vi "Main Tclk.vi"() -> ()   [LabVIEW 2018] (continued)
                        n3579 = local read "BD1 high limit array"() -> (w9160:sgl[])
                        n3580 = local read "Beam Dump 1 (nA)"() -> (w9152:sgl)
                        n3581 = local read "BD1 low limit array"() -> (w9156:sgl[])
                        n3582 = In Range and Coerce(upper limit=w9153, x=w9152, lower limit=w9154) -> (In Range?=w9163:bool)  [unwired: 1 out]
                        n3583 = Build Array (concatenate)(w9160, w9153) -> (w9158:sgl[])
                        n3584 = Build Array (concatenate)(w9156, w9154) -> (w9157:sgl[])
                        n3585 = Not(x=w9163) -> (.not. x?=w9162:bool)
                        n3586 = local write "BD1 high limit array"(w9158) -> ()
                        n3587 = local write "BD1 low limit array"(w9157) -> ()
                      }
                      frame 2 {
                        n3588 = Add(x=w9164, y=w9174) -> (x+y=w9172:sgl)
                        n3589 = Subtract(x=w9174, y=w9164) -> (x-y=w9168:sgl)
                        n3590 = To Single Precision Float(number=w9172) -> (single precision float=w9166:sgl)
                        n3591 = To Single Precision Float(number=w9168) -> (single precision float=w9167:sgl)
                        n3592 = local read "BD2 high limit array"() -> (w9173:sgl[])
                        n3593 = local read "Beam Dump 2 (nA)"() -> (w9165:sgl)
                        n3594 = local read "BD2 low limit array"() -> (w9169:sgl[])
                        n3595 = In Range and Coerce(upper limit=w9166, x=w9165, lower limit=w9167) -> (In Range?=w9176:bool)  [unwired: 1 out]
                        n3596 = Build Array (concatenate)(w9173, w9166) -> (w9171:sgl[])
                        n3597 = Build Array (concatenate)(w9169, w9167) -> (w9170:sgl[])
                        n3598 = Not(x=w9176) -> (.not. x?=w9175:bool)
                        n3599 = local write "BD2 high limit array"(w9171) -> ()
                        n3600 = local write "BD2 low limit array"(w9170) -> ()
                      }
                      frame 3 {
                        n3601 = Add(x=w9177, y=w9187) -> (x+y=w9185:sgl)
                        n3602 = Subtract(x=w9187, y=w9177) -> (x-y=w9181:sgl)
                        n3603 = To Single Precision Float(number=w9185) -> (single precision float=w9179:sgl)
                        n3604 = To Single Precision Float(number=w9181) -> (single precision float=w9180:sgl)
                        n3605 = local read "Milling I high limit array"() -> (w9186:sgl[])
                        n3606 = local read "Milling I (nA)"() -> (w9178:sgl)
                        n3607 = local read "Milling I low limit array"() -> (w9182:sgl[])
                        n3608 = In Range and Coerce(upper limit=w9179, x=w9178, lower limit=w9180) -> (In Range?=w9189:bool)  [unwired: 1 out]
                        n3609 = Build Array (concatenate)(w9186, w9179) -> (w9184:sgl[])
                        n3610 = Build Array (concatenate)(w9182, w9180) -> (w9183:sgl[])
                        n3611 = Not(x=w9189) -> (.not. x?=w9188:bool)
                        n3612 = local write "Milling I high limit array"(w9184) -> ()
                        n3613 = local write "Milling I low limit array"(w9183) -> ()
                      }
                      frame 100, Default {
                      }
                    }
                  }
                }
                n3614 = case shown="True" w9087 {
                  tunnel: w9086 -> [_ w9131]
                  tunnel: [FALSE w9130] -> w9085
                  frame False {
                  }
                  frame True {
                    n3615 = local read "Faraday Cup (nA)"() -> (w9132:sgl)
                    n3616 = Greater?(x=w9131, y=w9132) -> (0:w9130:bool)
                  }
                }
                "Faraday Cup < Milling current" <- w9085
                n3617 = case shown="True" w9114 {
                  tunnel: w9113 -> [_ w9204]
                  tunnel: w9106 -> [w9198 w9205]
                  tunnel: [w9198 w9199] -> _
                  frame False {
                  }
                  frame True {
                    n3618 = call "Auto limits.vi"("Minimum half range"=0.8, "# of interquartile range or stdev"=4.0 ("# of sigma"), "Input array"=w9204) -> ("Low limit"=w9202:dbl, "High limit"=w9203:dbl)  [unwired: 6 in, 1 out]
                    n3619 = Bundle By Name(cluster=w9205, "High limit (F)"=w9203, "Low limit (F)"=w9202) -> (w9199:T36)
                    n3620 = local write "Alert Settings"(w9199) -> ()
                  }
                }
                n3621 = Divide(x=w9045, y=w9048) -> (x/y=w9030:dbl)
                n3622 = Greater Or Equal?(x=w9095, y=w9109) -> (x >= y?=w9110:bool)
                n3623 = Round Toward +Infinity(x=w9030) -> (ceil(x): smallest int >= x=w9031:dbl)
                n3624 = Greater Or Equal?(x=sgl 1e-06, y=w9095) -> (x >= y?=w9052:bool)
                n3625 = To Unsigned Byte Integer(number=w9031) -> (unsigned 8bit integer=w9046:u8)
                n3626 = case shown="False" w9110 {
                  tunnel: w9112 -> [w9196 _]
                  tunnel: w9052 -> [w9194 _]
                  tunnel: [w9191 w9197] -> w9032
                  frame False {
                    n3627 = Select(t=u8 2 ("FI below limit counts"), s=w9194, f=u8 1 ("FI below limit counts")) -> (s? t:f=w9195:u8)
                    n3628 = Add(x=w9196, y=w9195) -> (x+y=w9191:u8)
                    n3629 = local write "FI below limit counts"(w9191) -> ()
                  }
                  frame True {
                    w9197 = u8 0 ("FI below limit counts")
                    n3630 = local write "FI below limit counts"(w9197) -> ()
                  }
                }
                n3631 = Less Or Equal?(x=w9046, y=w9032) -> (x <= y?=w9053:bool)
                n3632 = And(x=w9111, y=w9053) -> (x .and. y?=→"Focus index stop trigger active":bool)
                n3633 = Multiply(x=w9046, y=w9048) -> (x*y=→"Z removal stop threshold Z(nm)":dbl)
                n3634 = local read "Beam Dump 1 (nA)"() -> (w9107:sgl)
                n3635 = local read "Faraday Cup (nA)"() -> (w9100:sgl)
                n3636 = expression code="abs(x*0.05)"(w9100) -> (w9057:sgl)
                n3637 = In Range and Coerce(upper limit=sgl 1.0, x=w9057, lower limit=sgl 0.0) -> (coerced(x)=w9054:sgl)  [unwired: 1 out]
                n3638 = local read "FIB CL I out of bound counts"() -> (w9033:u8)
                n3639 = Less Or Equal?(x=w9107, y=w9054) -> (x <= y?=w9098:bool)
                n3640 = Less Or Equal?(x=w9100, y=sgl 0.1) -> (x <= y?=w9097:bool)
                n3641 = local read "Milling para"() -> (w9039:T35)
                n3642 = local read "Est. cycle time (s)"() -> (w9059:u32)
                n3643 = local read "SEM Specimen I array"() -> (w9082:sgl[])
                n3644 = local read "SEM Specimen I"() -> (w9075:dbl)
                n3645 = Or(x=w9098, y=w9097) -> (x .or. y?=→"Beam dump at zero":bool)
                n3646 = local read "Alert Settings"() -> (w9061:T36)
                n3647 = Unbundle By Name(w9039) -> ("Line milling time (s)"=w9038:sgl, "Lines auto pause"=w9037:u16)
                n3648 = local read "SEM Specimen I low limit array"() -> (w9074:sgl[])
                n3649 = local read "SEM Specimen I high limit array"() -> (w9071:sgl[])
                n3650 = expression code="21600/x"(w9059) -> (w9058:u32)
                n3651 = Increment(x=w9033) -> (x+1=w9104:u8)
                n3652 = call "Auto limits.vi"("Minimum half range"=0.1, "# of interquartile range or stdev"=4.0 ("# of sigma"), "Length"=w9058, "Input array"=w9082) -> ("Low limit"=w9073:dbl, "High limit"=w9070:dbl)  [unwired: 5 in, 1 out]
                n3653 = Unbundle By Name(w9061) -> ("Specimen @ SEM alarm"=w9060:bool)
                n3654 = Select(t=w9104, s=w9103, f=u8 0 ("y")) -> (s? t:f=w9040:u8)
                n3655 = Multiply(x=w9038, y=w9037) -> (x*y=w9036:sgl)
                n3656 = To Single Precision Float(number=w9070) -> (single precision float=w9068:sgl)
                n3657 = To Single Precision Float(number=w9073) -> (single precision float=w9067:sgl)
                n3658 = local write "FIB CL I out of bound counts"(w9040) -> ()
                n3659 = Greater?(x=w9036, y=sgl 6.0) -> (0:w9034:bool)
                n3660 = Build Array (concatenate)(w9074, w9067) -> (w9072:sgl[])
                n3661 = Build Array (concatenate)(w9071, w9068) -> (w9069:sgl[])
                n3662 = Select(t=w9040, s=w9034, f=w9033) -> (s? t:f=w9041:u8)
                n3663 = In Range and Coerce(upper limit=w9068, x=w9075, lower limit=w9067) -> (In Range?=w9081:bool)  [unwired: 1 out]
                n3664 = Greater Or Equal?(x=w9041, y=w9046) -> (x >= y?=→"FIB CL I alarm active":bool)
                n3665 = local write "SEM Specimen I low limit array"(w9072) -> ()
                n3666 = local write "SEM Specimen I high limit array"(w9069) -> ()
                n3667 = Not(x=w9081) -> (.not. x?=w9063:bool)
                n3668 = And(x=w9063, y=w9060) -> (x .and. y?=→"SEM Spec. I spike":bool)
              }
              frame #41 {
                n3669 = local read "Total progress"() -> (w9241:u8)
                n3670 = local read "Milling para"() -> (w9229:T35)
                n3671 = local read "FIB"() -> (w9208:bool)
                n3672 = local read "Alert Settings"() -> (w9209:T36)
                n3673 = Unbundle By Name(w9209) -> ("FIB emission warning"=w9207:bool)
                n3674 = local read "Alert Settings"() -> (w9217:T36)
                n3675 = local read "SW error warning active"() -> (w9215:bool)
                n3676 = Equal?(x=w9241, y=u8 100) -> (x = y?=w9240:bool)
                n3677 = And(x=w9208, y=w9207) -> (x .and. y?=w9206:bool)
                n3678 = Unbundle By Name(w9209) -> ("High limit (F)"=w9235:sgl, "Low limit (F)"=w9234:sgl, "Pause 3D-ING"=w9230:bool)  [unwired: 1 out]
                n3679 = Unbundle By Name(w9217) -> ("SW error warning"=w9216:bool)
                n3680 = case shown="False" w9240 {
                  tunnel: [w9326 FALSE ("Initialization")] -> w9237
                  frame False {
                    n3681 = local read "Machine Type"() -> (w9325:u8)
                    n3682 = case shown="2" w9325 {
                      tunnel: [w9329 w9341] -> w9326
                      frame 0, Default {
                        n3683 = local read "Hardware Configuration"() -> (w9328:T25)
                        n3684 = Unbundle By Name(w9328) -> ("Eanable COM"=w9327:bool)
                        n3685 = case shown="True" w9327 {
                          tunnel: [FALSE w9337] -> w9329
                          frame False {
                          }
                          frame True {
                            w9335 = TRUE ("Initialization")
                            n3686 = local read "COM port"() -> (w9336:refnum<visa-resource-name>)
                            n3687 = call "Remcon32 command.vi"("Close session"=w9335, "Initialization"=w9335, "SEM command"="eht?", "COM port in"=w9336) -> ("SEM reply"=w9333:string)  [unwired: 4 in, 3 out]
                            n3688 = Fract/Exp String To Number(string=w9333, default (0 dbl)=sgl 0.0 ("value (0)")) -> (number=w9331:sgl)  [unwired: 3 out]
                            n3689 = Equal To 0?(x=w9331) -> (x = 0?=w9337:bool)
                            "EHT off" <- w9337
                          }
                        }
                      }
                      frame 2 {
                        n3690 = local read "Api"() -> (w9338:refnum<k7>)
                        n3691 = call "SmartSEM Remote API get float.vi"("lpszParam"="AP_ACTUALKV", "Api"=w9338) -> ("vValue"=w9340:sgl)  [unwired: 7 in, 2 out]
                        n3692 = Equal To 0?(x=w9340) -> (x = 0?=w9341:bool)
                        n3693 = local write "EHT off"(w9341) -> ()
                      }
                    }
                  }
                  frame True {
                    w9344 = FALSE ("FIB")
                    n3694 = local write "FIB"(w9344) -> ()
                    n3695 = local write "3D FIB-SEM"(w9344) -> ()
                    n3696 = local write "Mill Stop"(TRUE ("Initialization")) -> ()
                    n3697 = local read "Machine Type"() -> (w9346:u8)
                    n3698 = local write "Status message"("3D FIB-SEM Completed" ("Status message")) -> ()
                    n3699 = case shown="2" w9346 {
                      frame 0, Default {
                      }
                      frame 1 {
                        n3700 = stacked-sequence {
                          frame #0 {
                            w9348 = FALSE ("Mill")
                            n3701 = local write "Mill"(w9348) -> ()
                            n3702 = local write "Mill Stop"(TRUE ("Rect Milling Stop")) -> ()
                            n3703 = local write "Mill Manual Pause"(w9348) -> ()
                          }
                          frame #1 {
                            w9350 = TRUE ("Initialization")
                            n3704 = local read "COM port"() -> (w9356:refnum<visa-resource-name>)
                            n3705 = call "FIB mode.vi"("Initialization"=w9350, "FIB mode"=T10."SEM", "COM port in"=w9356) -> ("COM port out"=w9355:refnum<visa-resource-name>)  [unwired: 7 in, 1 out]
                            n3706 = call "Remcon32 command.vi"("SEM command"="edx 0", "COM port in"=w9355) -> ("COM port out"=w9354:refnum<visa-resource-name>)  [unwired: 6 in, 3 out]
                            n3707 = call "Remcon32 command.vi"("Close session"=w9350, "SEM command"="frez", "COM port in"=w9354) -> ()  [unwired: 5 in, 4 out]
                          }
                        }
                      }
                      frame 2 {
                        n3708 = local read "Api"() -> (w9361:refnum<k7>)
                        n3709 = call "SmartSEM Remote API FIB mode.vi"("FIB mode"=T50."SEM", "Api"=w9361) -> ("error out"=w9357:errorcluster, "Api out"=w9358:refnum<k7>)  [unwired: 8 in]
                        n3710 = invoke class="_EMApi" method="Execute"(reference=w9358, error in=w9357, "lpszCommand"="CMD_FREEZE_ALL") -> ()  [unwired: 1 in, 4 out]
                      }
                    }
                    n3711 = local read "Email recipents file"() -> (w9342:path)
                    n3712 = Delete(path (use dialog)=w9342) -> ()  [unwired: 4 in, 3 out]
                  }
                }
                n3713 = case shown="True" w9206 {
                  tunnel: [FALSE w9282] -> w9218
                  tunnel: w9229 -> [_ w9301]
                  frame False {
                  }
                  frame True {
                    w9281 = u8 0 ("f")
                    n3714 = local read "FIB emission below limit counts"() -> (w9292:u8)
                    n3715 = local read "FIB suppressor below limit counts"() -> (w9286:u8)
                    n3716 = Unbundle By Name(w9301) -> ("Suppressor (V)"=w9294:sgl, "Emission (uA)"=w9295:dbl)
                    n3717 = local read "Machine Type"() -> (w9302:u8)
                    n3718 = local read "Alert Settings"() -> (w9306:T36)
                    n3719 = case shown="2" w9302 {
                      tunnel: [w9311 w9315 w9323] -> w9303
                      tunnel: w9295 -> [w9309 w9316 w9322]
                      tunnel: [w9310 w9314 w9319] -> w9291
                      tunnel: w9294 -> [_ _ w9320]
                      tunnel: [FALSE FALSE w9318] -> w9287
                      frame 0, Default {
                        n3720 = local read "HV Data Output"() -> (w9312:T18)
                        n3721 = Unbundle By Name(w9312) -> ("Emission (uA)"=w9311:sgl)
                        n3722 = Greater Or Equal?(x=w9309, y=w9311) -> (x >= y?=w9310:bool)
                      }
                      frame 1 {
                        n3723 = local read "FIB Parameters"() -> (w9317:T19)
                        n3724 = Unbundle By Name(w9317) -> ("FIB emission (uA)"=w9315:sgl)
                        n3725 = Greater Or Equal?(x=w9316, y=w9315) -> (x >= y?=w9314:bool)
                      }
                      frame 2 {
                        n3726 = local read "Capella HV Data Output"() -> (w9324:T17)
                        n3727 = Unbundle By Name(w9324) -> ("Suppressor (V)"=w9321:sgl, "Emission Actual (uA)"=w9323:sgl)
                        n3728 = Greater Or Equal?(x=w9322, y=w9323) -> (x >= y?=w9319:bool)
                        n3729 = Greater Or Equal?(x=w9320, y=w9321) -> (x >= y?=w9318:bool)
                      }
                    }
                    n3730 = Unbundle By Name(w9306) -> ("High limit"=w9305:dbl, "Low limit"=w9304:dbl)
                    n3731 = In Range and Coerce(upper limit=w9305, x=w9303, lower limit=w9304) -> (In Range?=w9280:bool)  [unwired: 1 out]
                    n3732 = Increment(x=w9292) -> (x+1=w9293:u8)
                    n3733 = Increment(x=w9286) -> (x+1=w9288:u8)
                    n3734 = Not(x=w9280) -> (.not. x?=→"FIB emission limit warning active":bool)
                    n3735 = Select(t=w9293, s=w9291, f=w9281) -> (s? t:f=w9290:u8)
                    n3736 = Select(t=w9288, s=w9287, f=w9281) -> (s? t:f=w9289:u8)
                    n3737 = local write "FIB emission limit warning armed"(w9280) -> ()
                    n3738 = local write "FIB emission below limit counts"(w9290) -> ()
                    n3739 = local write "FIB suppressor below limit counts"(w9289) -> ()
                    n3740 = local read "Est. cycle time (s)"() -> (w9299:u32)
                    n3741 = Quotient & Remainder(x=u32 300, y=w9299) -> (floor(x/y)=w9298:u32)  [unwired: 1 out]
                    n3742 = In Range and Coerce(upper limit=u32 10, x=w9298, lower limit=u32 2 ("x")) -> (coerced(x)=w9285:u32)  [unwired: 1 out]
                    n3743 = Greater Or Equal?(x=w9292, y=w9285) -> (x >= y?=w9283:bool)
                    n3744 = Greater Or Equal?(x=w9286, y=w9285) -> (x >= y?=w9284:bool)
                    n3745 = Or(x=w9283, y=w9284) -> (x .or. y?=w9282:bool)
                  }
                }
                n3746 = local read "Temp (F)"() -> (w9236:sgl)
                n3747 = And(x=w9216, y=w9215) -> (x .and. y?=w9214:bool)
                n3748 = In Range and Coerce(upper limit=w9235, x=w9236, lower limit=w9234) -> (In Range?=w9233:bool)  [unwired: 1 out]
                "Temperature recovery active" <- w9233
                n3749 = Not(x=w9233) -> (.not. x?=w9232:bool)
                "Temperature warning active" <- w9232
                n3750 = And(x=w9232, y=w9230) -> (x .and. y?=w9231:bool)
                n3751 = local read "Faraday Cup < Milling current"() -> (w9220:bool)
                n3752 = local read "Focus index stop trigger active"() -> (w9228:bool)
                n3753 = local read "FIB CL I alarm active"() -> (w9222:bool)
                n3754 = local read "Alert Settings"() -> (w9227:T36)
                n3755 = local read "Beam dump at zero"() -> (w9224:bool)
                n3756 = Unbundle By Name(w9227) -> ("FIB CL current alarm"=w9223:bool, "Beam Dump 1 alarm"=w9225:bool)
                n3757 = local read "Milling Z voltage spike"() -> (w9219:bool)
                n3758 = local read "SEM Spec. I spike"() -> (w9221:bool)
                n3759 = And(x=w9222, y=w9223) -> (x .and. y?=w9212:bool)
                n3760 = And(x=w9225, y=w9224) -> (x .and. y?=w9226:bool)
                n3761 = Compound Arithmetic op=OR(w9237, w9218, w9231, w9228, w9212, w9226, w9221, w9220, w9219, w9214) -> (w9238:bool)
                n3762 = local read "Machine Type"() -> (w9210:u8)
                n3763 = case shown="0, Default" w9210 {
                  tunnel: [w9242 FALSE FALSE] -> w9213
                  frame 0, Default {
                    n3764 = local read "HV Data Output"() -> (w9247:T18)
                    n3765 = Unbundle By Name(w9247) -> ("Suppressor (V)"=w9246:sgl)
                    n3766 = local read "Faraday cup I low"() -> (w9243:bool)
                    n3767 = Greater Or Equal?(x=sgl -1800.0, y=w9246) -> (x >= y?=w9244:bool)
                    n3768 = Or(x=w9244, y=w9243) -> (x .or. y?=w9242:bool)
                  }
                  frame 1 {
                  }
                  frame 2 {
                  }
                }
                n3769 = And(x=w9212, y=w9213) -> (x .and. y?=w9211:bool)
                n3770 = case shown="True" w9238 {
                  tunnel: w9218 -> [_ w9253]
                  tunnel: w9211 -> [_ w9254]
                  frame False {
                  }
                  frame True {
                    w9255 = TRUE ("Rect Mill Manual Pause")
                    n3771 = Or(x=w9253, y=w9254) -> (x .or. y?=w9252:bool)
                    n3772 = local read "Milling para"() -> (w9257:T35)
                    n3773 = local read "Last good FI"() -> (w9269:sgl)
                    n3774 = local read "SEM Scan Parameters"() -> (w9267:T26)
                    n3775 = shared-variable ".\\Zeiss Library.lvlib\\Timestamp"() -> (w9272:timestamp)  [unwired: 1 in, 1 out]
                    n3776 = local write "Pause for reheat"(w9255) -> ()
                    n3777 = local write "3D image paused active"(w9255) -> ()
                    n3778 = local write "Mill Manual Pause"(w9255) -> ()
                    n3779 = local read "Re-engage Files"() -> (w9258:path)
                    n3780 = Unbundle By Name(w9257) -> ("Auto reheat"=w9250:bool, "FIB PID target"=w9256:sgl)
                    n3781 = local write "Pre-reheat FI"(w9269) -> ()
                    n3782 = local write "Config Tabs"(T24."FIB Milling" ("Config Tabs")) -> ()
                    n3783 = local write "Pre-reheat time"(w9272) -> ()
                    n3784 = Unbundle By Name(w9267) -> ("X center (um)"=w9270:sgl, "Y center (um)"=w9271:sgl, "Y stig"=w9265:sgl[][])
                    n3785 = Build Path(base path=w9258, name or relative path="pre.png " ("command line")) -> (appended path=w9263:path)
                    n3786 = And(x=w9252, y=w9250) -> (x .and. y?=w9266:bool)
                    n3787 = local read "3D FIB-SEM Files"() -> (w9261:path)
                    n3788 = case shown="True" w9266 {
                      tunnel: w9256 -> [_ w9274]
                      frame False {
                      }
                      frame True {
                        w9278 = TRUE ("Request to reheat")
                        n3789 = local read "Reheat Output"() -> (w9277:T21)
                        n3790 = local write "Start Reheat"(w9278) -> ()
                        n3791 = Bundle By Name(cluster=w9277, "Reheat Success"=FALSE) -> (w9276:T21)
                        n3792 = local write "Reheat Output"(w9276) -> ()
                        "Auto reheat running" <- w9278
                        "Pre-reheat FIB PID target" <- w9274
                      }
                    }
                    n3793 = local write "Pre-reheat X center (um)"(w9270) -> ()
                    n3794 = local write "Pre-reheat Y center (um)"(w9271) -> ()
                    n3795 = local write "Pre-reheat Y stig"(w9265) -> ()
                    n3796 = local write "Status message"("Paused" ("Status message")) -> ()
                    n3797 = Build Path(base path=w9261, name or relative path="LG low res.png " ("command line")) -> (appended path=w9262:path)
                    n3798 = property on="Mill Manual Pause" class="Bool (strict)"("DisabledEnum"=T44."Disabled and Grayed Out" ("Disabled")) -> ()  [unwired: 2 in, 2 out]
                    n3799 = Copy(9:TRUE ("run minimized? (F)"), 10:w9263, 11:w9262) -> ()  [unwired: 2 in, 3 out]
                  }
                }
              }
              frame #42 {
                w9401 = FALSE ("Rect Milling Line Paused")
                w9394 = TRUE ("Rect Milling Resume")
                n3800 = local read "FIB"() -> (w9396:bool)
                n3801 = local read "Initial Options"() -> (w9397:T27)
                n3802 = local read "FIB slice #"() -> (w9403:u32)
                n3803 = local read "FIB HW Config"() -> (w9400:T23)
                n3804 = shared-variable "My Computer\\Zeiss Library.lvlib\\Milling Resume"(w9394) -> ()  [unwired: 1 in, 1 out]
                n3805 = shared-variable "My Computer\\Zeiss Library.lvlib\\Milling Line Paused"(w9401) -> ()  [unwired: 1 in, 1 out]
                n3806 = local write "Reset Focus"(w9401) -> ()
                n3807 = case shown="False" w9396 {
                  frame False {
                    n3808 = local read "Machine Type"() -> (w9421:u8)
                    n3809 = local write "Mill"(FALSE ("Mill")) -> ()
                    n3810 = local write "Mill Stop"(TRUE ("Rect Milling Stop")) -> ()
                    n3811 = case shown="2" w9421 {
                      frame 0, Default {
                      }
                      frame 1 {
                        n3812 = stacked-sequence {
                          frame #0 {
                            n3813 = Wait (ms)(milliseconds to wait=u32 1000) -> ()  [unwired: 1 out]
                          }
                          frame #1 {
                            w9423 = TRUE ("Initialization")
                            n3814 = local read "COM port"() -> (w9429:refnum<visa-resource-name>)
                            n3815 = call "FIB mode.vi"("Initialization"=w9423, "FIB mode"=T10."SEM", "COM port in"=w9429) -> ("COM port out"=w9428:refnum<visa-resource-name>)  [unwired: 7 in, 1 out]
                            n3816 = call "Remcon32 command.vi"("SEM command"="edx 0", "COM port in"=w9428) -> ("COM port out"=w9427:refnum<visa-resource-name>)  [unwired: 6 in, 3 out]
                            n3817 = call "Remcon32 command.vi"("Close session"=w9423, "SEM command"="frez", "COM port in"=w9427) -> ()  [unwired: 5 in, 4 out]
                          }
                        }
                      }
                      frame 2 {
                        n3818 = local read "Api"() -> (w9434:refnum<k7>)
                        n3819 = call "SmartSEM Remote API FIB mode.vi"("FIB mode"=T50."SEM", "Api"=w9434) -> ("error out"=w9430:errorcluster, "Api out"=w9431:refnum<k7>)  [unwired: 8 in]
                        n3820 = invoke class="_EMApi" method="Execute"(reference=w9431, error in=w9430, "lpszCommand"="CMD_FREEZE_ALL") -> ()  [unwired: 1 in, 4 out]
                      }
                    }
                    n3821 = local read "Post #1up"() -> (w9418:tag)
                    n3822 = local read "Post #1down"() -> (w9417:tag)
                    n3823 = local read "Post #2up"() -> (w9419:tag)
                    n3824 = local read "Post #2down"() -> (w9420:tag)
                    n3825 = call "SEM shutter.vi"("Shutter close"=FALSE, "Shutter AO4"=w9420, "Shutter AO3"=w9419, "Shutter AO2"=w9417, "Shutter AO1"=w9418) -> ()  [unwired: 6 in, 1 out]
                  }
                  frame True {
                  }
                }
                n3826 = Increment(x=w9403) -> (x+1=w9402:u32)
                n3827 = Unbundle By Name(w9400) -> ("FIB Ext Scan"=w9398:tag)
                n3828 = local write "SEM Options"(w9397) -> ()
                n3829 = local write "FIB slice #"(w9402) -> ()
                n3830 = call "FIB ext scan.vi"("Ext on"=FALSE ("data"), "FIB Ext Scan"=w9398) -> ()  [unwired: 9 in, 1 out]
                n3831 = local read "Milling para"() -> (w9365:T35)
                n3832 = Bundle By Name(cluster=w9365, "FIB PID reset"=w9394) -> (w9395:T35)
                n3833 = shared-variable ".\\Zeiss Library.lvlib\\FIB PID reset"(w9394) -> ()  [unwired: 1 in, 1 out]
                n3834 = Unbundle By Name(w9365) -> ("FIB PID measured"=w9362:u8, "FIB PID target"=w9363:sgl)
                n3835 = local read "Specimen I (nA)"() -> (w9364:sgl)
                n3836 = local write "Milling para"(w9395) -> ()
                n3837 = case shown="0, Default" w9362 {
                  tunnel: w9364 -> [_ w9413]
                  tunnel: w9363 -> [_ w9409]
                  frame 0, Default {
                    n3838 = local read "Milling I (nA)"() -> (w9404:sgl)
                    n3839 = local write "FIB mill target by spec. I (nA)"(w9404) -> ()
                  }
                  frame 4 {
                    n3840 = Subtract(x=w9409, y=w9413) -> (x-y=w9412:sgl)
                    n3841 = Sign(1:w9409) -> (0:w9408:sgl)
                    n3842 = Sign(1:w9412) -> (0:w9411:sgl)
                    n3843 = Compound Arithmetic op=MULTIPLY(sgl 0.01 ("x"), w9408, w9411) -> (w9407:sgl)
                    n3844 = Add(x=w9407, y="FIB mill target by spec. I (nA)") -> (x+y=w9405:sgl)
                    n3845 = local write "FIB mill target by spec. I (nA)"(w9405) -> ()
                  }
                }
                n3846 = local read "SEM Scan Parameters"() -> (w9381:T26)
                n3847 = local read "WD Stig Aln tile offsets"() -> (w9375:T3)
                n3848 = Unbundle By Name(w9381) -> ("WD (mm)"=w9385:sgl[][], "X stig"=w9387:sgl[][], "Y stig"=w9390:sgl[][], "X aln"=w9391:sgl[][], "Y aln"=w9393:sgl[][], "dX (um)"=w9373:sgl[], "dY (um)"=w9368:sgl[], "Y tiles"=w9382:u8, "X tiles"=w9383:u8)
                n3849 = expression code="(x-1)/2"(w9382) -> (w9370:u8)
                n3850 = expression code="(x-1)/2"(w9383) -> (w9367:u8)
                n3851 = Index Array(array=w9385, index (row)=w9370, index (col)=w9367) -> (element=w9384:sgl)
                n3852 = Index Array(array=w9387, index (row)=w9370, index (col)=w9367) -> (element=w9386:sgl)
                n3853 = Index Array(array=w9390, index (row)=w9370, index (col)=w9367) -> (element=w9389:sgl)
                n3854 = Index Array(array=w9391, index (row)=w9370, index (col)=w9367) -> (element=w9388:sgl)
                n3855 = Index Array(array=w9393, index (row)=w9370, index (col)=w9367) -> (element=w9392:sgl)
                n3856 = Index Array(array=w9373, index=w9370) -> (element=w9372:sgl)
                n3857 = Index Array(array=w9368, index=w9367) -> (element=w9369:sgl)
                n3858 = Subtract(x=w9385, y=w9384) -> (x-y=w9380:sgl[][])
                n3859 = Subtract(x=w9387, y=w9386) -> (x-y=w9379:sgl[][])
                n3860 = Subtract(x=w9390, y=w9389) -> (x-y=w9378:sgl[][])
                n3861 = Subtract(x=w9391, y=w9388) -> (x-y=w9377:sgl[][])
                n3862 = Subtract(x=w9393, y=w9392) -> (x-y=w9376:sgl[][])
                n3863 = Subtract(x=w9373, y=w9372) -> (x-y=w9371:sgl[])
                n3864 = Subtract(x=w9368, y=w9369) -> (x-y=w9366:sgl[])
                n3865 = Bundle By Name(cluster=w9375, "dWD"=w9380, "dX stig"=w9379, "dY stig"=w9378, "dX aln"=w9377, "dY aln"=w9376, "dX (um)"=w9371, "dY (um)"=w9366) -> (w9374:T3)
                n3866 = local write "WD Stig Aln tile offsets"(w9374) -> ()
              }
            }
          }
        }
        n3867 = Wait Until Next ms Multiple(millisecond multiple=u32 100) -> ()  [unwired: 1 out]
      }
      n3868 = Open VI Reference(vi path=w710) -> (vi reference=w715:refnum<vi>, error out=w709:errorcluster)  [unwired: 1 in, 4 out]
      n3869 = register-events(error in=w709, refnum<vi> refnum) -> (reference out=w712:refnum<event-registration>)  [unwired: 1 in, 1 out]
      n3870 = local read "Trapezoidal"() -> (w707:cluster{"X":i16, "Y":i16}[])
      n3871 = while {
        tunnel: w712 -> [w2956]
        tunnel: [w2955] -> w713
        tunnel: [w2953] -> w714
        tunnel: w715 -> [w2954]
        shift-right: [w2948] -> _
        shift-left: w707 -> [w2947]
        stop <- w2952 stop-if-true
        n3872 = Wait Until Next ms Multiple(millisecond multiple=u32 1) -> ()  [unwired: 1 out]
        n3873 = event shown="[30] \"SEM Shutter\": Value Change" {
          selector: w2956 -> [_ _ _ _ _ _ _ _ _ _ _ _ _ _ _ _ _ _ _ _ _ _ _ _ _ _ _ w3658 _ w3861 _ _ _ _ _ _ _ _ _ _ _ _ _ _ _ _ _ _ _ _ _ _ _ _ _ _ _ _ _ _ _ _ _ _ _ _ _ _ _ _ _ _ _ _ _ _ _ _ _ _ _ _ _ _ _ _ _]
          dyn-events: [_ _ _ _ _ _ _ _ _ _ _ _ _ _ _ _ _ _ _ _ _ _ _ _ _ _ _ w3657 _ w3860 _ _ _ _ _ _ _ _ _ _ _ _ _ _ _ _ _ _ _ _ _ _ _ _ _ _ _ _ _ _ _ _ _ _ _ _ _ _ _ _ _ _ _ _ _ _ _ _ _ _ _ _ _ _ _ _ _] -> w2955
          timeout: _ -> [_ _ _ _ _ _ _ _ _ _ _ _ _ _ _ _ _ _ _ _ _ _ _ _ _ _ _ _ _ _ _ _ _ _ _ _ _ _ _ _ _ _ _ _ _ _ _ _ _ _ _ _ _ _ _ _ _ _ _ _ _ _ _ _ _ _ _ _ _ _ _ _ _ _ _ _ _ _ _ _ _ _ _ _ _ _ _]
          tunnel: [_ _ _ _ _ _ _ _ _ _ _ _ _ _ _ _ _ _ _ _ _ _ _ _ _ _ _ w3656 _ w3859 _ _ _ _ _ _ _ _ _ _ _ _ _ _ _ _ _ _ _ _ _ _ _ _ _ _ _ _ _ _ _ _ _ _ _ _ _ _ _ _ _ _ _ _ _ _ _ _ _ _ _ _ _ _ _ _ _] -> w2953
          tunnel: w2954 -> [_ _ _ _ _ _ _ _ _ _ _ _ _ _ _ _ _ _ _ _ _ _ _ _ _ _ _ w3654 _ _ _ _ _ _ _ _ _ _ _ _ _ _ _ _ _ _ _ _ _ _ _ _ _ _ _ _ _ _ _ _ _ _ _ _ _ _ _ _ _ _ _ _ _ _ _ _ _ _ _ _ _ _ _ _ _ _ _]
          tunnel: [_ _ _ _ _ _ _ _ _ w3222 _ _ _ _ _ _ _ _ _ _ _ _ _ _ _ _ _ _ _ _ _ _ _ _ _ _ _ _ _ _ _ _ _ _ _ _ _ _ _ _ _ _ _ _ _ _ _ _ _ _ _ _ _ _ _ _ _ _ _ _ _ _ _ _ _ _ _ _ _ _ _ _ _ _ _ _ _] -> w2950
          tunnel: [_ _ _ _ _ _ _ _ _ _ _ _ _ _ _ _ _ _ _ _ _ _ _ _ _ _ _ w3650 w3669 w3825 _ _ w3982 _ _ _ _ _ _ _ _ w4458 _ _ _ _ _ _ _ _ _ _ _ _ _ _ _ _ _ _ _ _ _ _ _ _ _ _ _ _ _ _ _ _ _ _ _ _ _ _ _ _ _ _ _ _ _] -> w2948
          tunnel: w2947 -> [_ _ _ _ _ _ _ _ _ _ _ _ _ _ _ _ _ _ _ _ _ _ _ _ _ _ _ w3650 w3668 w3825 _ _ _ _ _ _ _ _ _ _ _ w4457 _ _ _ _ _ _ _ _ _ _ _ _ _ _ _ _ _ _ _ _ _ _ _ _ _ _ _ _ _ _ _ _ _ _ _ _ _ _ _ _ _ _ _ _ _]
          event Timeout {
            n3874 = event-data() -> ()  [unwired: 3 out]
          }
          event Key Down? {
            # "Ignore Ctrl-W, Alt-F4"
            n3875 = event-data() -> ("Char"=w2968:i16, "VKey"=w2965:T48, "PlatMods"=w2963:T77)  [unwired: 7 out]
            n3876 = Unbundle By Name(w2963) -> ("Ctrl"=w2962:bool, "Alt"=w2960:bool)
            n3877 = Equal?(x=w2968, y=i16 119) -> (x = y?=w2966:bool)
            n3878 = Equal?(x=w2965, y=eventvkey."F4" ("VKey")) -> (x = y?=w2961:bool)
            n3879 = And(x=w2966, y=w2962) -> (x .and. y?=w2959:bool)
            n3880 = And(x=w2960, y=w2961) -> (x .and. y?=w2958:bool)
            n3881 = Compound Arithmetic op=OR(w2959, w2958) -> (w2957:bool)
            n3882 = event-data("Discard?"=w2957) -> ()  [unwired: 6 in, 1 out]
          }
          event "Scan x1": Value Change {
            n3883 = event-data() -> ()  [unwired: 6 out]
          }
          event "3D FIB-SEM": Value Change {
            n3884 = event-data() -> ("NewVal"=w2969:bool)  [unwired: 5 out]
            n3885 = case shown="True" w2969 {
              frame False {
                n3886 = Two Button Dialog(message="Stop 3D FIB-SEM?") -> (T button?=w2970:bool)  [unwired: 2 in]
                n3887 = local write "Mill Stop"(w2970) -> ()
                n3888 = case shown="True" w2970 {
                  frame False {
                    n3889 = local write "3D FIB-SEM"(TRUE ("3D FIB-SEM")) -> ()
                  }
                  frame True {
                    n3890 = stacked-sequence {
                      frame #0 {
                        n3891 = shared-variable "My Computer\\Zeiss Library.lvlib\\Milling Stop"(TRUE ("Milling Stop")) -> ()  [unwired: 1 in, 1 out]
                        n3892 = Wait (ms)(milliseconds to wait=u32 1000) -> ()  [unwired: 1 out]
                      }
                      frame #1 {
                        w2975 = FALSE ("3D FIB-SEM")
                        n3893 = local read "Last FIB recipe"() -> (w2985:path)
                        n3894 = local read "Email recipents file"() -> (w2979:path)
                        n3895 = local read "FIB Image"() -> (w2990:i16[][])
                        n3896 = Array Size(array=w2990) -> (size(s)=w2989:i32[])
                        n3897 = local write "Pause for reheat"(w2975) -> ()
                        n3898 = local write "3D FIB-SEM"(w2975) -> ()
                        n3899 = local write "FIB"(w2975) -> ()
                        n3900 = Add Array Elements(numeric array=w2989) -> (sum=w2988:i32)
                        n3901 = Not Equal To 0?(x=w2988) -> (x != 0?=w2987:bool)
                        n3902 = Open/Create/Replace File(file path (use dialog)=w2985) -> (error out=w2983:errorcluster)  [unwired: 5 in, 2 out]
                        n3903 = case shown="True" w2987 {
                          tunnel: w2990 -> [_ w3016]
                          frame False {
                          }
                          frame True {
                            n3904 = local read "Last FIB image"() -> (w3019:path)
                            n3905 = call "16bit Image Normalization.vi"("Transpose"=FALSE, "Input image"=w3016) -> ("Normalized image"=w3015:u8[][])  [unwired: 5 in, 4 out]
                            n3906 = call <vilib>:"Flatten Pixmap.vi"("colors"=u32[] [16777222, 65793, 131586, 197379, 263172, 328965, 394758, 460551, 526344, 592137, 657930, 723723, 789516, 855309, 921102, 986895, 1052688, 1118481, 1184274, 1250067, 1315860, 1381653, 1447446, 1513239, 1579032, 1644825, 1710618, 1776411, 1842204, 1907997, 1973790, 2039583, 2105376, 2171169, 2236962, 2302755, 2368548, 2434341, 2500134, 2565927, 2631720, 2697513, 2763306, 2829099, 2894892, 2960685, 3026478, 3092271, 3158064, 3223857, 3289650, 3355443, 3421236, 3487029, 3552822, 3618615, 3684408, 3750201, 3815994, 3881787, 3947580, 4013373, 4079166, 4144959, 4210752, 4276545, 4342338, 4408131, 4473924, 4539717, 4605510, 4671303, 4737096, 4802889, 4868682, 4934475, 5000268, 5066061, 5131854, 5197647, 5263440, 5329233, 5395026, 5460819, 5526612, 5592405, 5658198, 5723991, 5789784, 5855577, 5921370, 5987163, 6052956, 6118749, 6184542, 6250335, 6316128, 6381921, 6447714, 6513507, 6579300, 6645093, 6710886, 6776679, 6842472, 6908265, 6974058, 7039851, 7105644, 7171437, 7237230, 7303023, 7368816, 7434609, 7500402, 7566195, 7631988, 7697781, 7763574, 7829367, 7895160, 7960953, 8026746, 8092539, 8158332, 8224125, 8289918, 8355711, 8421504, 8487297, 8553090, 8618883, 8684676, 8750469, 8816262, 8882055, 8947848, 9013641, 9079434, 9145227, 9211020, 9276813, 9342606, 9408399, 9474192, 9539985, 9605778, 9671571, 9737364, 9803157, 9868950, 9934743, 10000536, 10066329, 10132122, 10197915, 10263708, 10329501, 10395294, 10461087, 10526880, 10592673, 10658466, 10724259, 10790052, 10855845, 10921638, 10987431, 11053224, 11119017, 11184810, 11250603, 11316396, 11382189, 11447982, 11513775, 11579568, 11645361, 11711154, 11776947, 11842740, 11908533, 11974326, 12040119, 12105912, 12171705, 12237498, 12303291, 12369084, 12434877, 12500670, 12566463, 12632256, 12698049, 12763842, 12829635, 12895428, 12961221, 13027014, 13092807, 13158600, 13224393, 13290186, 13355979, 13421772, 13487565, 13553358, 13619151, 13684944, 13750737, 13816530, 13882323, 13948116, 14013909, 14079702, 14145495, 14211288, 14277081, 14342874, 14408667, 14474460, 14540253, 14606046, 14671839, 14737632, 14803425, 14869218, 14935011, 15000804, 15066597, 15132390, 15198183, 15263976, 15329769, 15395562, 15461355, 15527148, 15592941, 15658734, 15724527, 15790320, 15856113, 15921906, 15987699, 16053492, 16119285, 16185078, 16250871, 16316664, 16382457, 16448250, 16514043, 16579836, 16645629, 16711422, 16448250] ("256 gray scale"), "8-bit pixmap"=w3015) -> ("image data"=w3018:T55)  [unwired: 4 in, 5 out]
                            n3907 = call <vilib>:"Write PNG File.vi"("image data"=w3018, "path to PNG file"=w3019) -> ()  [unwired: 1 in, 9 out]
                          }
                        }
                        n3908 = File/Directory Info(path=w2979) -> (path out=w2976:path, error out=w2978:errorcluster)  [unwired: 1 in, 5 out]
                        n3909 = Unbundle By Name(w2983) -> ("status"=w2984:bool)
                        n3910 = Unbundle By Name(w2978) -> ("status"=w2977:bool)
                        n3911 = local read "Recipe input"() -> (w2981:T7)
                        n3912 = case shown="False" w2984 {
                          tunnel: w2985 -> [w3013 w3014]
                          tunnel: [w3012 w3014] -> w2982
                          frame False {
                            n3913 = Delete(path (use dialog)=w3013) -> (deleted path=w3012:path)  [unwired: 4 in, 2 out]
                          }
                          frame True {
                          }
                        }
                        n3914 = case shown="False" w2977 {
                          tunnel: w2976 -> [w2999 _]
                          frame False {
                            n3915 = Delete(path (use dialog)=w2999) -> ()  [unwired: 4 in, 3 out]
                          }
                          frame True {
                          }
                        }
                        n3916 = call "Recipe read write.vi"("Write"=TRUE, "Recipe path"=w2982, "Write input"=w2981) -> ()  [unwired: 5 in, 4 out]
                        n3917 = local read "Detector A Low Mag"() -> (w2992:i16[][])
                        n3918 = local read "Detector B Low Mag"() -> (w2991:i16[][])
                        n3919 = Array Size(array=w2992) -> (size(s)=w2993:i32[])
                        n3920 = Array Size(array=w2991) -> (size(s)=w2998:i32[])
                        n3921 = Add Array Elements(numeric array=w2993) -> (sum=w2994:i32)
                        n3922 = Add Array Elements(numeric array=w2998) -> (sum=w2997:i32)
                        n3923 = Not Equal To 0?(x=w2994) -> (x != 0?=w2995:bool)
                        n3924 = Not Equal To 0?(x=w2997) -> (x != 0?=w2996:bool)
                        n3925 = case shown="True" w2995 {
                          tunnel: w2992 -> [_ w3008]
                          frame False {
                          }
                          frame True {
                            n3926 = local read "Last Det A Low Mag"() -> (w3010:path)
                            n3927 = call "16bit Image Normalization.vi"("Transpose"=FALSE, "Input image"=w3008) -> ("Normalized image"=w3007:u8[][])  [unwired: 5 in, 4 out]
                            n3928 = call <vilib>:"Flatten Pixmap.vi"("colors"=u32[] [16777222, 65793, 131586, 197379, 263172, 328965, 394758, 460551, 526344, 592137, 657930, 723723, 789516, 855309, 921102, 986895, 1052688, 1118481, 1184274, 1250067, 1315860, 1381653, 1447446, 1513239, 1579032, 1644825, 1710618, 1776411, 1842204, 1907997, 1973790, 2039583, 2105376, 2171169, 2236962, 2302755, 2368548, 2434341, 2500134, 2565927, 2631720, 2697513, 2763306, 2829099, 2894892, 2960685, 3026478, 3092271, 3158064, 3223857, 3289650, 3355443, 3421236, 3487029, 3552822, 3618615, 3684408, 3750201, 3815994, 3881787, 3947580, 4013373, 4079166, 4144959, 4210752, 4276545, 4342338, 4408131, 4473924, 4539717, 4605510, 4671303, 4737096, 4802889, 4868682, 4934475, 5000268, 5066061, 5131854, 5197647, 5263440, 5329233, 5395026, 5460819, 5526612, 5592405, 5658198, 5723991, 5789784, 5855577, 5921370, 5987163, 6052956, 6118749, 6184542, 6250335, 6316128, 6381921, 6447714, 6513507, 6579300, 6645093, 6710886, 6776679, 6842472, 6908265, 6974058, 7039851, 7105644, 7171437, 7237230, 7303023, 7368816, 7434609, 7500402, 7566195, 7631988, 7697781, 7763574, 7829367, 7895160, 7960953, 8026746, 8092539, 8158332, 8224125, 8289918, 8355711, 8421504, 8487297, 8553090, 8618883, 8684676, 8750469, 8816262, 8882055, 8947848, 9013641, 9079434, 9145227, 9211020, 9276813, 9342606, 9408399, 9474192, 9539985, 9605778, 9671571, 9737364, 9803157, 9868950, 9934743, 10000536, 10066329, 10132122, 10197915, 10263708, 10329501, 10395294, 10461087, 10526880, 10592673, 10658466, 10724259, 10790052, 10855845, 10921638, 10987431, 11053224, 11119017, 11184810, 11250603, 11316396, 11382189, 11447982, 11513775, 11579568, 11645361, 11711154, 11776947, 11842740, 11908533, 11974326, 12040119, 12105912, 12171705, 12237498, 12303291, 12369084, 12434877, 12500670, 12566463, 12632256, 12698049, 12763842, 12829635, 12895428, 12961221, 13027014, 13092807, 13158600, 13224393, 13290186, 13355979, 13421772, 13487565, 13553358, 13619151, 13684944, 13750737, 13816530, 13882323, 13948116, 14013909, 14079702, 14145495, 14211288, 14277081, 14342874, 14408667, 14474460, 14540253, 14606046, 14671839, 14737632, 14803425, 14869218, 14935011, 15000804, 15066597, 15132390, 15198183, 15263976, 15329769, 15395562, 15461355, 15527148, 15592941, 15658734, 15724527, 15790320, 15856113, 15921906, 15987699, 16053492, 16119285, 16185078, 16250871, 16316664, 16382457, 16448250, 16514043, 16579836, 16645629, 16711422, 16448250] ("256 gray scale"), "8-bit pixmap"=w3007) -> ("image data"=w3009:T55)  [unwired: 4 in, 5 out]
                            n3929 = call <vilib>:"Write PNG File.vi"("image data"=w3009, "path to PNG file"=w3010) -> ()  [unwired: 1 in, 9 out]
                          }
                        }
                        n3930 = case shown="True" w2996 {
                          tunnel: w2991 -> [_ w3001]
                          frame False {
                          }
                          frame True {
                            n3931 = local read "Last Det B Low Mag"() -> (w3004:path)
                            n3932 = call "16bit Image Normalization.vi"("Transpose"=FALSE, "Input image"=w3001) -> ("Normalized image"=w3000:u8[][])  [unwired: 5 in, 4 out]
                            n3933 = call <vilib>:"Flatten Pixmap.vi"("colors"=u32[] [16777222, 65793, 131586, 197379, 263172, 328965, 394758, 460551, 526344, 592137, 657930, 723723, 789516, 855309, 921102, 986895, 1052688, 1118481, 1184274, 1250067, 1315860, 1381653, 1447446, 1513239, 1579032, 1644825, 1710618, 1776411, 1842204, 1907997, 1973790, 2039583, 2105376, 2171169, 2236962, 2302755, 2368548, 2434341, 2500134, 2565927, 2631720, 2697513, 2763306, 2829099, 2894892, 2960685, 3026478, 3092271, 3158064, 3223857, 3289650, 3355443, 3421236, 3487029, 3552822, 3618615, 3684408, 3750201, 3815994, 3881787, 3947580, 4013373, 4079166, 4144959, 4210752, 4276545, 4342338, 4408131, 4473924, 4539717, 4605510, 4671303, 4737096, 4802889, 4868682, 4934475, 5000268, 5066061, 5131854, 5197647, 5263440, 5329233, 5395026, 5460819, 5526612, 5592405, 5658198, 5723991, 5789784, 5855577, 5921370, 5987163, 6052956, 6118749, 6184542, 6250335, 6316128, 6381921, 6447714, 6513507, 6579300, 6645093, 6710886, 6776679, 6842472, 6908265, 6974058, 7039851, 7105644, 7171437, 7237230, 7303023, 7368816, 7434609, 7500402, 7566195, 7631988, 7697781, 7763574, 7829367, 7895160, 7960953, 8026746, 8092539, 8158332, 8224125, 8289918, 8355711, 8421504, 8487297, 8553090, 8618883, 8684676, 8750469, 8816262, 8882055, 8947848, 9013641, 9079434, 9145227, 9211020, 9276813, 9342606, 9408399, 9474192, 9539985, 9605778, 9671571, 9737364, 9803157, 9868950, 9934743, 10000536, 10066329, 10132122, 10197915, 10263708, 10329501, 10395294, 10461087, 10526880, 10592673, 10658466, 10724259, 10790052, 10855845, 10921638, 10987431, 11053224, 11119017, 11184810, 11250603, 11316396, 11382189, 11447982, 11513775, 11579568, 11645361, 11711154, 11776947, 11842740, 11908533, 11974326, 12040119, 12105912, 12171705, 12237498, 12303291, 12369084, 12434877, 12500670, 12566463, 12632256, 12698049, 12763842, 12829635, 12895428, 12961221, 13027014, 13092807, 13158600, 13224393, 13290186, 13355979, 13421772, 13487565, 13553358, 13619151, 13684944, 13750737, 13816530, 13882323, 13948116, 14013909, 14079702, 14145495, 14211288, 14277081, 14342874, 14408667, 14474460, 14540253, 14606046, 14671839, 14737632, 14803425, 14869218, 14935011, 15000804, 15066597, 15132390, 15198183, 15263976, 15329769, 15395562, 15461355, 15527148, 15592941, 15658734, 15724527, 15790320, 15856113, 15921906, 15987699, 16053492, 16119285, 16185078, 16250871, 16316664, 16382457, 16448250, 16514043, 16579836, 16645629, 16711422, 16448250] ("256 gray scale"), "8-bit pixmap"=w3000) -> ("image data"=w3003:T55)  [unwired: 4 in, 5 out]
                            n3934 = call <vilib>:"Write PNG File.vi"("image data"=w3003, "path to PNG file"=w3004) -> ()  [unwired: 1 in, 9 out]
                          }
                        }
                        n3935 = property on="Pause for reheat" class="Bool (strict)"("DisabledEnum"=T44."Disabled and Grayed Out" ("Disabled")) -> ()  [unwired: 2 in, 2 out]
                      }
                    }
                  }
                }
              }
              frame True {
                n3936 = local read "Milling para"() -> (w3023:T35)
                n3937 = Unbundle By Name(w3023) -> ("Mill start from Last"=w3022:bool)
                n3938 = Two Button Dialog(message="Confirm FIB milling probe,\nand start 3D FIB-SEM?") -> (T button?=w3025:bool)  [unwired: 2 in]
                n3939 = And(x=w3025, y=w3022) -> (x .and. y?=w3026:bool)
                n3940 = local read "Machine Type"() -> (w3021:u8)
